vi "LIDAR-Test-On-cRIO.vi"() -> ()   [LabVIEW 2010]
uses:
  <vilib>/Platform/TimedLoop/XDataNode/XDataNode.xnode
  <vilib>/Platform/TimedLoop/XDataNode/timing_clust.ctl
  <vilib>/Platform/TimedLoop/XDataNode/nitl_modes.ctl
  <vilib>/Platform/TimedLoop/XDataNode/wakeup.ctl
  <instrlib>/Hokuyo URG Series/Public/Initialize-Standard.vi
  <instrlib>/Hokuyo URG Series/Hokuyo URG Series.lvlib
  <vilib>/Platform/TimedLoop/XDataNode/XDNodeRunTimeDep.lvlib
panel:
  out "Angle Array":dbl[](array[numeric])
  out "Magnitude Array":dbl[](array[numeric])
  in  "ID Query?":bool
  in  "VISA resource name":refnum<visa-resource-name>="TCPIP::10.10.10.15::10940::Socket"
  in  "Stop":bool
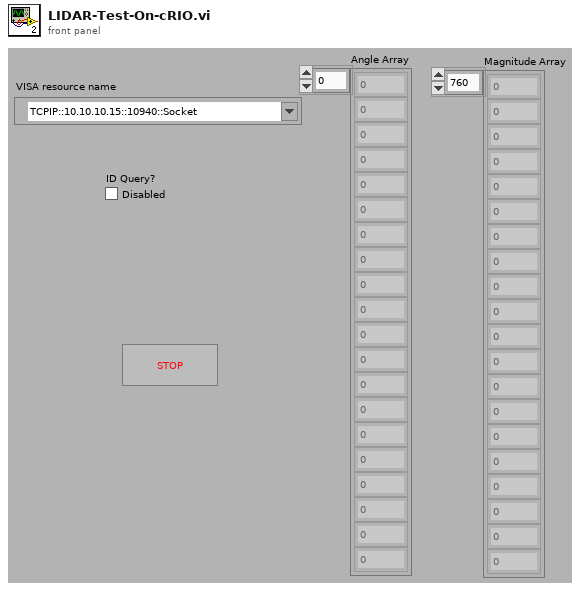
[diagram p1: front panel]
types:
  T1 = typedef "XDNodeRunTimeDep.lvlib/timing_clust.ctl" = cluster{"Expected End [f-1]":u64, "Actual End [f-1]":u64, "Finished Late? [f-1]":bool, "Expected End [i-1]":u64, "Actual End [i-1]":u64, "Finished Late? [i-1]":bool, "Expected Start [i]":u64, "Actual Start [i]":u64, "Expected Start [f]":u64, "Actual Start [f]":u64, "Source Name":string, "Structure Name":string, "Period":i64, "Deadline":i64, "Offset":i64, "Start":i64, "Priority":i32, "Timeout":i32, "Mode":T2, "Wakeup Reason":T3, "Error":errorcluster, "Source Type":string, "Secondary Source Type":string, "Global End Time":u64, "Global Start Time":u64, "Frame Duration":u64, "Iteration Duration":u64, "Assigned CPU":i32, "I/O Scan Engine Mode":u32}
  T2 = typedef "XDNodeRunTimeDep.lvlib/nitl_modes.ctl" = enum32{"No Change", "Process missed periods, maintain original phase", "Discard missed periods, maintain original phase", "Process missed periods, ignore original phase", "Discard missed periods, ignore original phase"}
  T3 = typedef "XDNodeRunTimeDep.lvlib/wakeup.ctl" = enum32{"Normal", "Aborted", "Asynchronous wakeup", "Timing source error", "Timed loop error", "Timeout"}
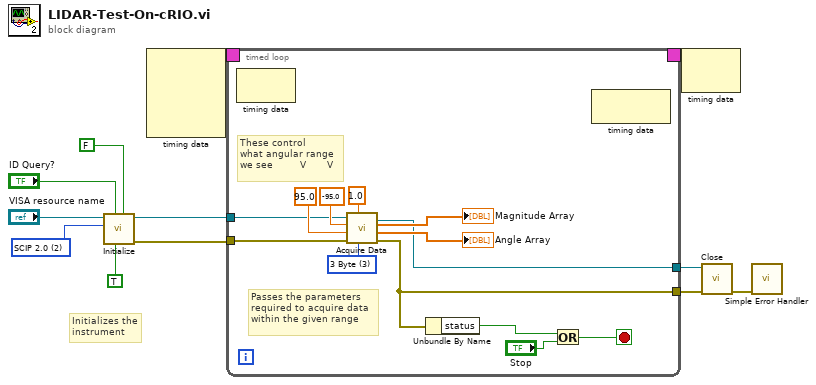
[diagram p0: block diagram]
diagram:
  w3 = u32 2 items=["Convert to Latest", "SCIP 1.1", "SCIP 2.0", "SCIP 2.2"] ("Protocol (2: SCIP 2.0)")
  # "Initializes the instrument"
  n1 = call-poly <instrlib>:"Initialize.vi"("Reset? (F: No)"=FALSE ("Reset Instrument (Disabled)"), "Checksum (Disabled)"=TRUE ("Checksum"), "ID Query? (Enabled)"="ID Query?", "Protocol (2: SCIP 2.0)"=w3, "VISA resource name"="VISA resource name") -> ("error out"=w4:errorcluster, "VISA resource name out"=w5:refnum<visa-resource-name>)  [unwired: 5 in]
  n2 = node-c288() -> (w2:T1)  [unwired: 4 in]
  n3 = timed-loop {
    tunnel: w5 -> [w17]
    tunnel: [w13] -> w12
    tunnel: [w14] -> w6
    tunnel: w4 -> [w16]
    timing: w2 -> [_]
    timing-out: [_] -> w1
    stop <- w23 stop-if-true
    w15 = u16 3 items=["2 Byte"=2, "3 Byte"=3] ("Encoding Width")
    # "These control\nwhat angular range\nwe see         V       V"
    # "Passes the parameters\nrequired to acquire data\nwithin the given range"
    n4 = node-c288() -> ()  [unwired: 1 in, 1 out]
    n5 = call <instrlib>:"Acquire Data.vi"("Data Encoding Width (3 Byte)"=w15, "Cluster Count (1)"=1.0 ("Cluster Count"), "error in (no error)"=w16, "End Point (120°)"=95.0 ("End Point"), "Start Point (-120°)"=-95.0 ("Start Point"), "VISA resource name"=w17) -> ("error out"=w13:errorcluster, "Direction"=→"Angle Array":dbl[], "Magnitude"=→"Magnitude Array":dbl[], "VISA resource name out"=w14:refnum<visa-resource-name>)  [unwired: 2 in]
    n6 = Unbundle By Name(w13) -> ("status"=w25:bool)
    n7 = Or(x=w25, y="Stop") -> (x .or. y?=w23:bool)
    n8 = node-c288() -> ()  [unwired: 1 in, 1 out]
  }
  n9 = node-c288(w1) -> ()  [unwired: 1 out]
  n10 = call <instrlib>:"Close.vi"("error in (no error)"=w12, "VISA resource name"=w6) -> ("error out"=w9:errorcluster)  [unwired: 9 in]
  n11 = call <vilib>:"Simple Error Handler.vi"("error in (no error)"=w9) -> ()  [unwired: 4 in, 5 out]
